vi "time string to minutes string.vi"(11 "Array":string[](array[string])) -> (3 "output string":string)   [LabVIEW 2017]
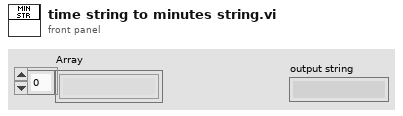
[diagram p1: front panel]
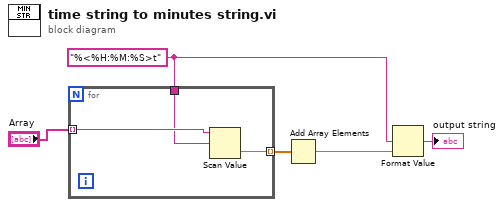
[diagram p0: block diagram]
diagram:
  w2 = "%<%H:%M:%S>t" ("format string")
  n1 = for {
    tunnel: "Array" -> [w8] mode=indexing
    tunnel: [w7] -> w4 mode=indexing
    tunnel: w2 -> [w6]
    n2 = Scan Value(string=w8, format string=w6) -> (value=w7:dbl)  [unwired: 1 in, 1 out]
  }
  n3 = Add Array Elements(numeric array=w4) -> (sum=w3:dbl)
  n4 = Format Value(format string=w2, value (0)=w3) -> (output string=→"output string":string)  [unwired: 1 in]
